vi "install.vi"(8 "error in (no error)":errorcluster, 11 "plugin_interface in":refnum<class "lv-post-installer-test.lvclass">=refnum) -> (0 "error out":errorcluster, 3 "plugin_interface out":refnum<class "lv-post-installer-test.lvclass">)   [LabVIEW 2015, in "lv-post-installer.lvlib" / "lv-post-installer-test.lvclass"]
uses:
  lv-post-installer-test.lvclass
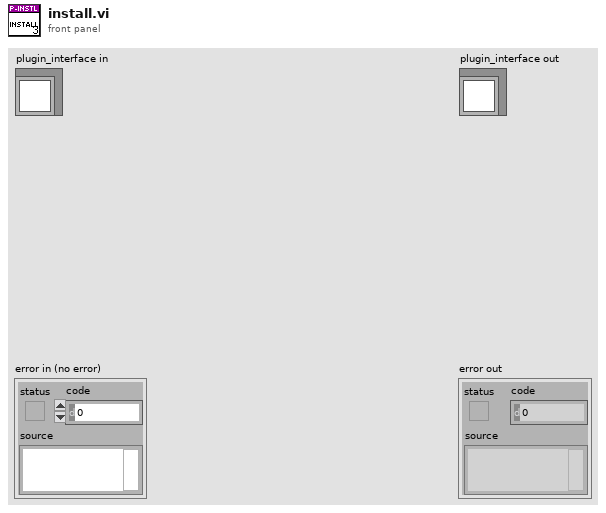
[diagram p1: front panel]
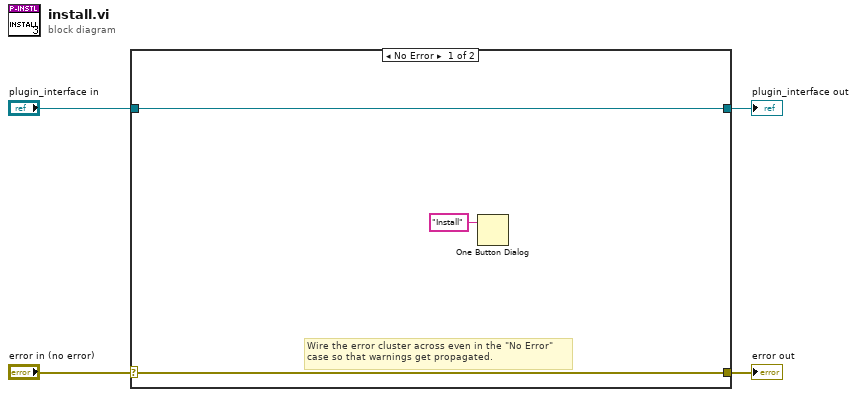
[diagram p0: block diagram]
diagram:
  n1 = case shown="No Error" "error in (no error)" {
    selector: "error in (no error)" -> [w6 w9]
    tunnel: [w6 w9] -> w3
    tunnel: [w7 w8] -> w1
    tunnel: "plugin_interface in" -> [w7 w8]
    frame No Error {
      # "Wire the error cluster across even in the \"No Error\"\ncase so that warnings get propagated."
      n2 = One Button Dialog(message="Install") -> ()  [unwired: 1 in, 1 out]
    }
    frame Error {
    }
  }
  "error out" <- w3
  "plugin_interface out" <- w1
